vi "P-541 Set Port.vi"(0 "VISA Ref In":refnum<visa-resource-name>, 11 "Error In":errorcluster) -> (4 "VISA Ref Out":refnum<visa-resource-name>, 15 "Error Out":errorcluster)   [LabVIEW 2020]
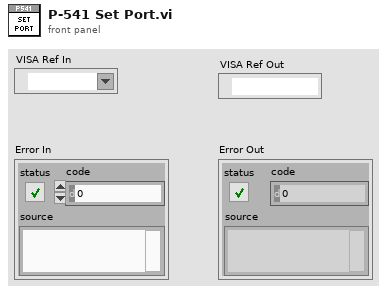
[diagram p1: front panel]
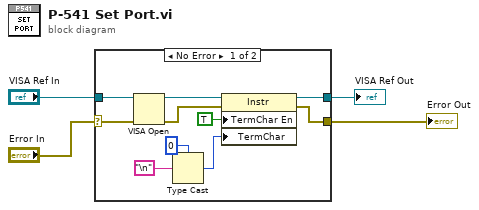
[diagram p0: block diagram]
diagram:
  n1 = case shown="No Error" "Error In" {
    selector: "Error In" -> [w6 w15]
    tunnel: "VISA Ref In" -> [w8 w16]
    tunnel: [w7 w16] -> w3
    tunnel: [w5 w15] -> w1
    frame No Error {
      n2 = VISA Open(error in (no error)=w6, VISA resource name=w8) -> (VISA resource name=w14:refnum<visa-resource-name>, error out=w9:errorcluster)  [unwired: 3 in]
      n3 = Type Cast(type=u8 0, x="\n") -> (*(type *) &x=w10:u8)
      n4 = property class="Instr"(reference=w14, error in=w9, "TermChar En"=TRUE ("Message Based Settings:Termination Character Enable"), "TermChar"=w10) -> (reference out=w7:refnum<visa-resource-name>, error out=w5:errorcluster)
    }
    frame Error {
    }
  }
  "VISA Ref Out" <- w3
  "Error Out" <- w1
